vi "QWTB Algorithms Filter Set List.vi"(10 "algs list":string[](array[string]), 11 "info data":string) -> (3 "info data out":string)   [LabVIEW 2020]
uses:
  octave/infolib/String.vi
  octave/infolib/1D String.vi
  octave/infolib/infolib.lvlib
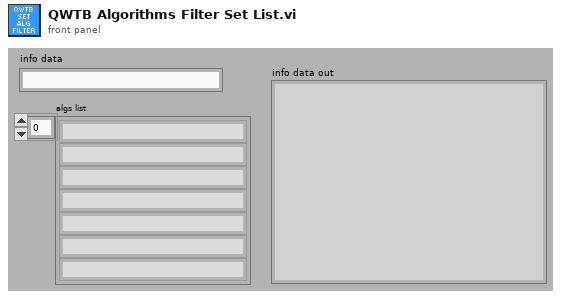
[diagram p1: front panel]
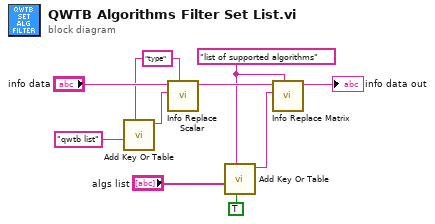
[diagram p0: block diagram]
diagram:
  w7 = "list of supported algorithms" ("key description")
  w3 = "type" ("key description")
  n1 = call-poly "Add Key Or Table.vi"("key description"=w3, "string"="qwtb list") -> ("info data out"=w2:string)  [unwired: 8 in, 1 out]
  n2 = call "Info Replace Scalar.vi"("key description to replace"=w3, "info data to paste"=w2, "info data in"="info data") -> ("info data out"=w9:string)  [unwired: 8 in]
  n3 = call-poly "Add Key Or Table.vi"("collumn vector (F)"=TRUE, "key description"=w7, "string"="algs list") -> ("info data out"=w6:string)  [unwired: 7 in, 1 out]
  n4 = call "Info Replace Matrix.vi"("key description to replace"=w7, "info data to paste"=w6, "info data in"=w9) -> ("info data out"=→"info data out":string)  [unwired: 8 in]
